vi "LucaDetectIon.vi"(8 "error in (no error)":errorcluster, 10 "Threshold":i32, 11 "array":u16[][](array[numeric])) -> (0 "error out":errorcluster, 1 "Counts":i32, 2 "Ion":bool, 3 "output array":u16[][](array[numeric]))   [LabVIEW 2009]
panel:
  out "Intensity Graph":u16[][](graph)
  in  "Acquisition Timeout":i32=1000
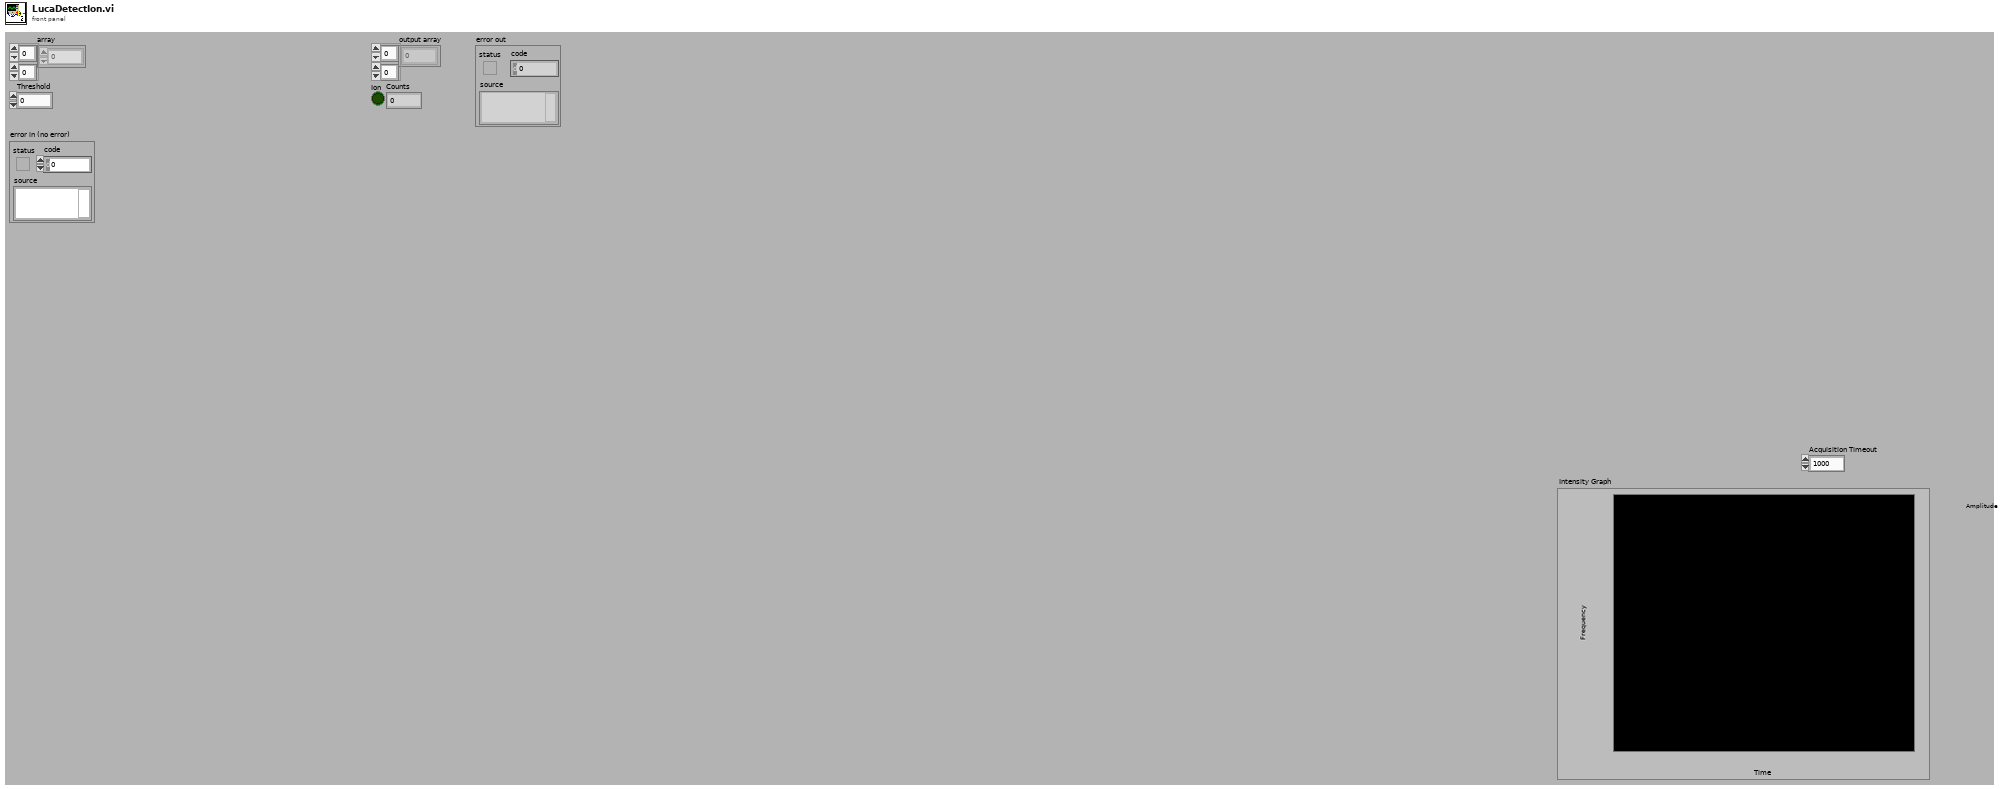
[diagram p1: front panel]
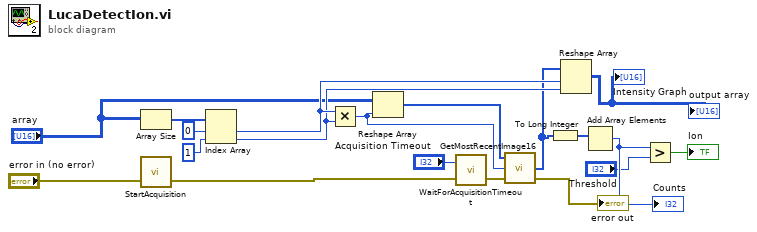
[diagram p0: block diagram]
diagram:
  n1 = Array Size(array="array") -> (size(s)=w18:i32[])
  n2 = call <userlib>:"StartAcquisition.vi"("error in (no error)"="error in (no error)") -> ("error out"=w19:errorcluster)  [unwired: 1 in, 1 out]
  n3 = Index Array(array=w18, index #1=0 ("index"), index #2=1 ("index")) -> (element #1=w15:i32, element #2=w14:i32)
  n4 = Multiply(x=w15, y=w14) -> (x*y=w8:i32)
  n5 = Reshape Array("array", w8) -> (w12:u16[])
  n6 = call <userlib>:"WaitForAcquisitionTimeout.vi"("error in (no error)"=w19, "iTimeOutMs"="Acquisition Timeout") -> ("error out"=w13:errorcluster)  [unwired: 1 out]
  n7 = call <userlib>:"GetMostRecentImage16.vi"("error in (no error)"=w13, "size"=w8, "array"=w12) -> ("error out"=→"error out":errorcluster, "array"=w2:u16[])  [unwired: 1 out]
  n8 = To Long Integer(number=w2) -> (32bit integer=w1:i32[])
  n9 = Reshape Array(w2, w15, w14) -> (→"Intensity Graph" →"output array":u16[][])
  n10 = Add Array Elements(numeric array=w1) -> (sum=w5:i32)
  "Counts" <- w5
  n11 = Greater?(x=w5, y="Threshold") -> (0:→"Ion":bool)
